vi "open calibration.vi"(7 "Index":u32) -> (2 "conversion out":T6={"conversion matrix"=[[0.0, 0.0], [0.0, 0.0], [0.0, 0.0], [0.0, 0.0], [0.0, 0.0], [0.0, 0.0]], "units"="", "name"="", "scale type"=enum."Volts", "offset (volts)"=0.0, "second channel"=0, "correspondence table"=[], "offset (physical units)"=0.0, "pH scale"={"Buffers"=[], "Temperature"=0.0}, "D.O."={"Temperature"=0.0, "K"=0.0, "barometric pressure"=0.0}} {"D.O."."K" format="%.6f"; "D.O."."Temperature" format="%.2f"; "pH scale"."Buffers"."V/T" format="%.5f"; "pH scale"."Buffers"."Buffer" format="%.2f"; "pH scale"."Temperature" format="%.2f"; "offset (physical units)" format="%.5f"; "correspondence table"."volts" format="%.4f"; "correspondence table"."physical units" format="%.4f"; "second channel" min=-1; "offset (volts)" format="%.5f"; "conversion matrix" format="%.4e"})   [LabVIEW 2012]
uses:
  calibration/conversion.ctl
  DAQ configuration/scale type.ctl
  calibration/correspondence table.ctl
  calibration/pH/pH scale.ctl
  calibration/Dissolved Oxygen/DO scale.ctl
  calibration/conversion 3.ctl
  DAC project/Calibration and Function folders.ctl
  calibration/global scale array.vi
panel:
  in  "conversion 3":T1={"conversion matrix"=[[0.0, 0.0], [0.0, 0.0], [0.0, 0.0], [0.0, 0.0], [0.0, 0.0], [0.0, 0.0]], "units"="", "name"="", "scale type"=enum."Volts", "offset (volts)"=0.0, "second channel"=0, "correspondence table"=[], "offset (physical units)"=0.0, "pH scale"={"Buffers"=[], "Temperature"=0.0}, "D.O."={"Temperature"=0.0, "K"=0.0}} {"D.O."."K" format="%.6f"; "D.O."."Temperature" format="%.2f"; "pH scale"."Buffers"."V/T" format="%.5f"; "pH scale"."Buffers"."Buffer" format="%.2f"; "pH scale"."Temperature" format="%.2f"; "offset (physical units)" format="%.5f"; "correspondence table"."volts" format="%.4f"; "correspondence table"."physical units" format="%.4f"; "second channel" min=-1; "offset (volts)" format="%.5f"; "conversion matrix" format="%.4e"}
  out "file age":i32
  in  "conversion 2":T4={"conversion matrix"=[[0.0, 0.0], [0.0, 0.0], [0.0, 0.0], [0.0, 0.0], [0.0, 0.0], [0.0, 0.0]], "units"="", "name"="", "scale type"=enum."Volts", "offset (volts)"=0.0, "second channel"=0, "correspondence table"=[], "offset (physical units)"=0.0} {"offset (physical units)" format="%.5f"; "correspondence table"."volts" format="%.4f"; "correspondence table"."physical units" format="%.4f"; "second channel" min=-1; "offset (volts)" format="%.5f"; "conversion matrix" format="%.4e"}
  in  "conversion 1":T5={"conversion matrix"=[[0.0, 0.0], [0.0, 0.0], [0.0, 0.0], [0.0, 0.0], [0.0, 0.0], [0.0, 0.0]], "units"="", "name"="", "scale type"=enum."Volts", "offset (volts)"=0.0, "second channel"=0, "correspondence table"=[], "offset (physical units)"=0.0} {"offset (physical units)" format="%.5f"; "correspondence table"."volts" format="%.4f"; "correspondence table"."physical units" format="%.4f"; "second channel" min=-1; "offset (volts)" format="%.5f"; "conversion matrix" format="%.4e"}
  # "C"
  # "C"
  # "C"
  # "kPa"
  # "C"
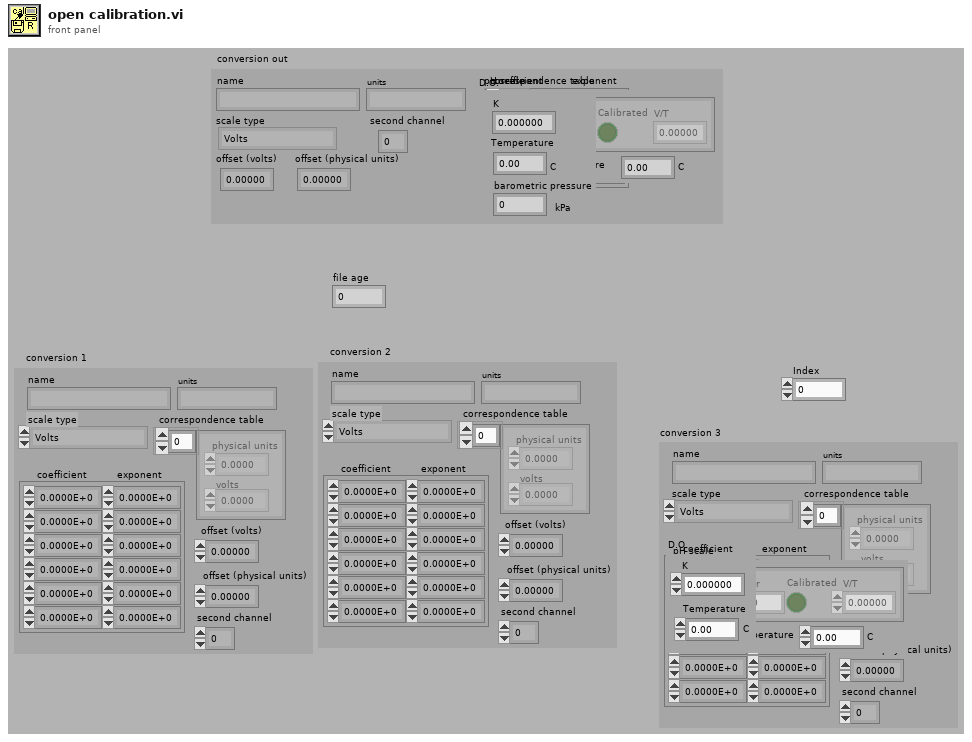
[diagram p1: front panel]
types:
  T1 = typedef "conversion 3.ctl" = cluster{"conversion matrix":sgl[][], "units":string, "name":string, "scale type":enum16{"Volts", "Polynomial", "Correspondence Table", "pH", "Dissolved Oxygen", "Quadratic"}, "offset (volts)":dbl, "second channel":i8, "correspondence table":cluster{"physical units":dbl, "volts":dbl}[], "offset (physical units)":dbl, "pH scale":cluster{"Buffers":cluster{"Buffer":dbl, "Calibrated":bool, "V/T":dbl}[], "Temperature":dbl}, "D.O.":cluster{"Temperature":dbl, "K":dbl}}
  T2 = typedef "scale type.ctl" = enum16{"Volts", "Polynomial", "Correspondence Table", "pH", "Dissolved Oxygen", "Quadratic"}
  T3 = typedef "correspondence table.ctl" = cluster{"physical units":dbl, "volts":dbl}[]
  T4 = cluster{"conversion matrix":sgl[][], "units":string, "name":string, "scale type":T2, "offset (volts)":dbl, "second channel":i8, "correspondence table":T3, "offset (physical units)":dbl}
  T5 = cluster{"conversion matrix":sgl[][], "units":string, "name":string, "scale type":enum16{"Volts", "Polynomial", "Correspondence Table", "pH", "Dissolved Oxygen"}, "offset (volts)":dbl, "second channel":i8, "correspondence table":T3, "offset (physical units)":dbl}
  T6 = typedef "conversion.ctl" = cluster{"conversion matrix":sgl[][], "units":string, "name":string, "scale type":T2, "offset (volts)":dbl, "second channel":i8, "correspondence table":T3, "offset (physical units)":dbl, "pH scale":T7, "D.O.":T8}
  T7 = typedef "pH scale.ctl" = cluster{"Buffers":cluster{"Buffer":dbl, "Calibrated":bool, "V/T":dbl}[], "Temperature":dbl}
  T8 = typedef "DO scale.ctl" = cluster{"Temperature":dbl, "K":dbl, "barometric pressure":dbl}
  T9 = typedef "Calibration and Function folders.ctl" = enum16{"Sensors", "Functions", "Config File", "UserAppFolder"}
  T10 = enum16{"open", "open or create", "create or replace", "create", "open (read only)"}
  T11 = typedef "calib array.ctl" = T6[]
  T12 = enum16{"read/write", "read-only", "write-only", "write-only (truncate)"}
  T13 = enum16{"Volts", "Polynomial", "Correspondence Table", "pH", "Dissolved Oxygen"}
  T14 = enum16{"Volts", "Polynomial", "Correspondence Table", "pH", "Dissolved Oxygen", "Quadratic"}
  T15 = cluster{"Buffers":cluster{"Buffer":dbl, "Calibrated":bool, "V/T":dbl}[], "Temperature":dbl}
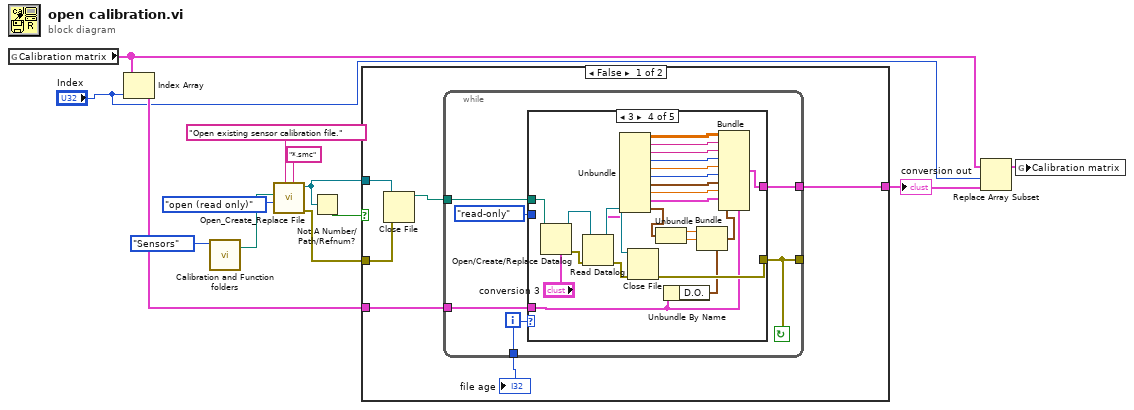
[diagram p0: block diagram]
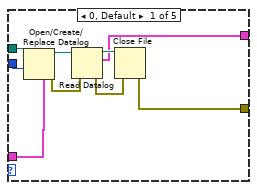
[diagram p2: hidden frame]
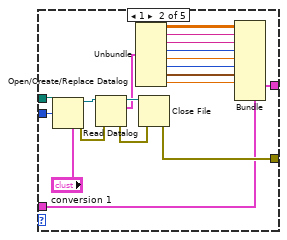
[diagram p3: hidden frame]
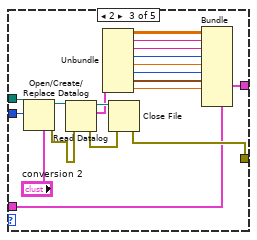
[diagram p4: hidden frame]
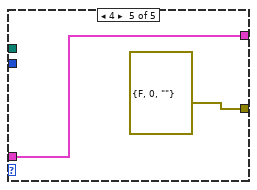
[diagram p5: hidden frame]
diagram:
  n1 = global read "global scale array.vi" "Calibration matrix"() -> (w5:T11)
  n2 = Index Array(array=w5, index="Index") -> (element=w7:T6)
  n3 = call "Calibration and Function folders.vi"("Folder"=Calibration_and_Function_folders."Sensors") -> ("Selected Folder"=w2:path)  [unwired: 10 in]
  n4 = call <vilib>:"Open_Create_Replace File.vi"("pattern"="*.smc", "prompt"="Open existing sensor calibration file.", "function (open:0)"=T10."open (read only)", "start path  (Not A Path)"=w2) -> ("error out"=w9:errorcluster, "refnum"=w8:refnum<file>)  [unwired: 4 in, 2 out]
  n5 = Not A Number/Path/Refnum?(number/path/refnum=w8) -> (NaN/Path/Refnum?=w10:bool)
  n6 = case shown="False" w10 {
    tunnel: w8 -> [w19 _]
    tunnel: w9 -> [w18 _]
    tunnel: [w16 w99] -> w6
    tunnel: w7 -> [w15 w99]
    frame False {
      n7 = Close File(refnum=w19, error in=w18) -> (path=w17:path)  [unwired: 1 out]
      n8 = while {
        tunnel: [w25] -> w14
        tunnel: w15 -> [w20]
        tunnel: [w21] -> w16
        tunnel: [w22] -> _
        tunnel: w17 -> [w23]
        i -> [w25]
        stop <- w22 continue-if-true
        n9 = case shown="3" w25 {
          tunnel: T12."read-only" ("open mode (0)") -> [w33 w52 w72 _ _]
          tunnel: w23 -> [w34 w53 w71 w85 _]
          tunnel: [w28 w46 w65 w81 errorcluster {"status"=FALSE, "code"=0, "source"=""} ("error out")] -> w22
          tunnel: [w27 w35 w62 w84 w97] -> w21
          tunnel: w20 -> [w26 w36 w63 w74 w97]
          frame 0, Default {
            n10 = Open/Create/Replace Datalog(5:w26, 9:w33, 11:w34) -> (0:w29:errorcluster, 3:w30:refnum<k1>)  [unwired: 3 in, 1 out]
            n11 = Read Datalog(4:w29, 7:w30) -> (0:w31:errorcluster, 2:w27:T6, 3:w32:refnum<k1>)  [unwired: 1 in]
            n12 = Close File(refnum=w32, error in=w31) -> (error out=w28:errorcluster)  [unwired: 1 out]
          }
          frame 1 {
            n13 = Open/Create/Replace Datalog(5:"conversion 1", 9:w52, 11:w53) -> (0:w48:errorcluster, 3:w47:refnum<k1>)  [unwired: 3 in, 1 out]
            n14 = Read Datalog(4:w48, 7:w47) -> (0:w49:errorcluster, 2:w37:T5, 3:w50:refnum<k1>)  [unwired: 1 in]
            n15 = Unbundle(w37) -> ("conversion matrix"=w45:sgl[][], "units"=w44:string, "name"=w43:string, "scale type"=w42:T13, "offset (volts)"=w41:dbl, "second channel"=w40:i8, "correspondence table"=w39:T3, "offset (physical units)"=w38:dbl)
            n16 = Close File(refnum=w50, error in=w49) -> (error out=w46:errorcluster)  [unwired: 1 out]
            n17 = Bundle(cluster=w36, "conversion matrix"=w45, "units"=w44, "name"=w43, "scale type"=w42, "offset (volts)"=w41, "second channel"=w40, "correspondence table"=w39, "offset (physical units)"=w38) -> (w35:T6)  [unwired: 2 in]
          }
          frame 2 {
            n18 = Open/Create/Replace Datalog(5:"conversion 2", 9:w72, 11:w71) -> (0:w68:errorcluster, 3:w69:refnum<k1>)  [unwired: 3 in, 1 out]
            n19 = Read Datalog(4:w68, 7:w69) -> (0:w66:errorcluster, 2:w64:T4, 3:w67:refnum<k1>)  [unwired: 1 in]
            n20 = Unbundle(w64) -> ("conversion matrix"=w61:sgl[][], "units"=w60:string, "name"=w59:string, "scale type"=w58:T2, "offset (volts)"=w57:dbl, "second channel"=w56:i8, "correspondence table"=w55:T3, "offset (physical units)"=w54:dbl)
            n21 = Close File(refnum=w67, error in=w66) -> (error out=w65:errorcluster)  [unwired: 1 out]
            n22 = Bundle(cluster=w63, "conversion matrix"=w61, "units"=w60, "name"=w59, "scale type"=w58, "offset (volts)"=w57, "second channel"=w56, "correspondence table"=w55, "offset (physical units)"=w54) -> (w62:T6)  [unwired: 2 in]
          }
          frame 3 {
            n23 = Open/Create/Replace Datalog(5:"conversion 3", 11:w85) -> (0:w83:errorcluster, 3:w96:refnum<k1>)  [unwired: 4 in, 1 out]
            n24 = Read Datalog(4:w83, 7:w96) -> (0:w82:errorcluster, 2:w94:T1, 3:w95:refnum<k1>)  [unwired: 1 in]
            n25 = Unbundle(w94) -> ("conversion matrix"=w93:sgl[][], "units"=w92:string, "name"=w91:string, "scale type"=w90:T14, "offset (volts)"=w89:dbl, "second channel"=w88:i8, "correspondence table"=w87:cluster{"physical units":dbl, "volts":dbl}[], "offset (physical units)"=w86:dbl, "pH scale"=w80:T15, "D.O."=w78:cluster{"Temperature":dbl, "K":dbl})
            n26 = Close File(refnum=w95, error in=w82) -> (error out=w81:errorcluster)  [unwired: 1 out]
            n27 = Unbundle(w78) -> ("Temperature"=w76:dbl, "K"=w75:dbl)
            n28 = Unbundle By Name(w74) -> ("D.O."=w73:T8)
            n29 = Bundle(cluster=w73, "Temperature"=w76, "K"=w75) -> (w77:T8)  [unwired: 1 in]
            n30 = Bundle(cluster=w74, "conversion matrix"=w93, "units"=w92, "name"=w91, "scale type"=w90, "offset (volts)"=w89, "second channel"=w88, "correspondence table"=w87, "offset (physical units)"=w86, "pH scale"=w80, "D.O."=w77) -> (w84:T6)
          }
          frame 4 {
          }
        }
      }
      "file age" <- w14
    }
    frame True {
    }
  }
  "conversion out" <- w6
  n31 = Replace Array Subset(array=w5, new element=w6, index="Index") -> (w3:T11)
  n32 = global write "global scale array.vi" "Calibration matrix"(w3) -> ()
